vi "VI server_Set Control Value from String Format.vi"(4 "Options":T1, 6 "Value.STR":string, 7 "Label":string, 8 "error in (no error)":errorcluster, 11 "VI Server Cluster":T2) -> (0 "error out":errorcluster, 3 "VI Server Cluster.DUP":T2)   [LabVIEW 2020, in "VI Server Toolkit LV2013.lvlib"]
doc: "Sets control to value formatted as strings."
uses:
  VI Server Toolkit LV2013.lvlib
  VI Server_TypeDefs/VI Server_RefsCluster.ctl
  VI Server Libraries/VI Server Controls.llb/VI Server_GetSet Controls From String Format_Options.ctl
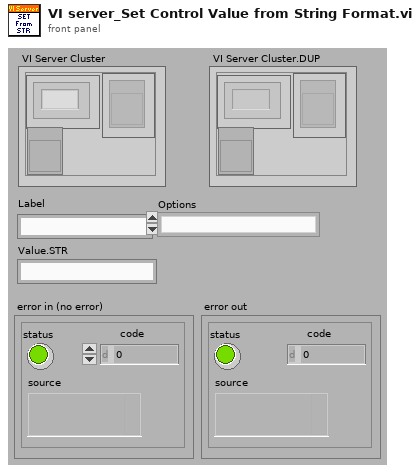
[diagram p1: front panel]
types:
  T1 = typedef "VI Server Toolkit LV2013.lvlib/VI Server_GetSet Controls From String Format_Options.ctl" = enum16{"", "If Ring Get Selection", "If Ring Set by Selection"}
  T2 = typedef "VI Server_RefsCluster.ctl" = cluster{"Labels":string[], "Refs":refnum<vi>[], "VI Ref":refnum<vi>}
  T3 = enum8{"Enabled", "Disabled", "Disabled and Grayed Out"}
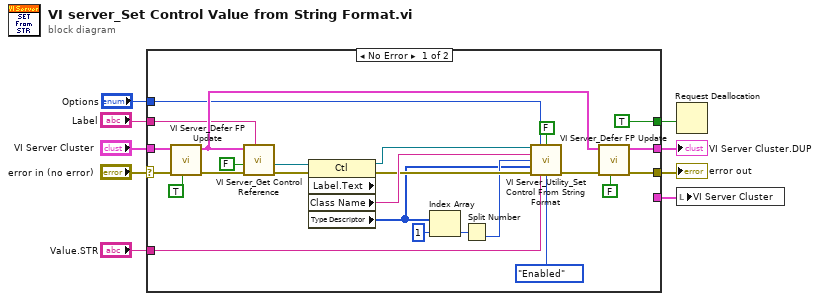
[diagram p0: block diagram]
diagram:
  n1 = case shown="No Error" "error in (no error)" {
    selector: "error in (no error)" -> [w29 w36]
    tunnel: "Label" -> [w13 _]
    tunnel: "Value.STR" -> [w30 _]
    tunnel: [w26 w36] -> w9
    tunnel: "VI Server Cluster" -> [w28 _]
    tunnel: [w23 _] -> w6
    tunnel: [TRUE _] -> w5
    tunnel: [_ w35] -> w4
    tunnel: "Options" -> [w10 _]
    frame No Error {
      n2 = call "VI Server_Defer FP Update.vi"("Defer Panel Updates? (F)"=TRUE ("Defer Panel Updates (F)"), "error in"=w29, "VI Server Cluster"=w28) -> ("error out"=w20:errorcluster, "VI Server Cluster.DUP"=w18:T2)  [unwired: 7 out]
      n3 = call "VI Server_Get Control Reference.vi"("Label"=w13, "error in"=w20, "Single Instance (T)"=FALSE, "VI Server Cluster"=w18) -> ("error out"=w19:errorcluster, "Control Reference (Generic)"=w14:refnum<vi>)  [unwired: 4 in, 2 out]
      n4 = property class="Ctl" props=["Label", "Text", "Class Name", "Type Descriptor"](reference=w14, error in=w19) -> (reference out=w34:refnum<vi>, error out=w32:errorcluster, "Class Name"=w33:string, "Type Descriptor"=w21:i16[])  [unwired: 1 out]
      n5 = Index Array(array=w21, index=1) -> (element=w15:i16)
      n6 = Split Number(x=w15) -> (lo(x)=w31:u8)  [unwired: 1 out]
      n7 = call "VI Server_Utility_Set Control From String Format.vi"("Control.Ref"=w34, "Options"=w10, 2:FALSE ("Option.Value(Signaling. F=Value)"), "ClassName"=w33, "Control.Representation"=w31, "TypeDesc"=w21, "error in (no error)"=w32, "Value.STR"=w30, 13:T3."Enabled" ("Disabled")) -> ("error out"=w25:errorcluster)  [unwired: 6 in]
      n8 = call "VI Server_Defer FP Update.vi"("Defer Panel Updates? (F)"=FALSE ("Defer Panel Updates (F)"), "error in"=w25, "VI Server Cluster"=w18) -> ("error out"=w26:errorcluster, "VI Server Cluster.DUP"=w23:T2)  [unwired: 7 out]
    }
    frame Error {
      n9 = call "VI Server_Empty VI Server Cluster.vi"() -> ("VI Server Cluster"=w35:T2)  [unwired: 7 in]
    }
  }
  "error out" <- w9
  "VI Server Cluster.DUP" <- w6
  n10 = Request Deallocation(w5) -> ()
  n11 = local write "VI Server Cluster"(w4) -> ()
